vi "Do Main Action.vi"(8 "error in (no error)":errorcluster, 10 "AbstractData":refnum<class "AbstractData.lvclass">, 11 "Pipelined Actor in":refnum<class "Pipelined Actor.lvclass">) -> (0 "error out":errorcluster, 3 "Pipelined Actor out":refnum<class "Pipelined Actor.lvclass">)   [LabVIEW 2014, in "Pipelined Actor.lvlib" / "Pipelined Actor.lvclass"]
uses:
  Pipelined Actor.lvclass
  Model/Data/AbstractData/AbstractData.lvclass
  Pipelined Actor.lvclass/Pipelined Actor.ctl
  <vilib>/ActorFramework/Message Enqueuer/Message Priority.ctl
  Pipelined Actor Messages/Do Main Action Msg/Do Main Action Msg.lvclass/Do Main Action Msg.ctl
  <vilib>/ActorFramework/Message Enqueuer/Message Enqueuer.lvclass/Message Enqueuer.ctl
  <vilib>/ActorFramework/Message Enqueuer/Enqueue.vi
  <vilib>/ActorFramework/Message Priority Queue/Priority Enqueue.vi
  <vilib>/ActorFramework/Message Enqueuer/Message Enqueuer.lvclass
  Pipelined Actor Messages/Do Main Action Msg/Do Main Action Msg.lvclass
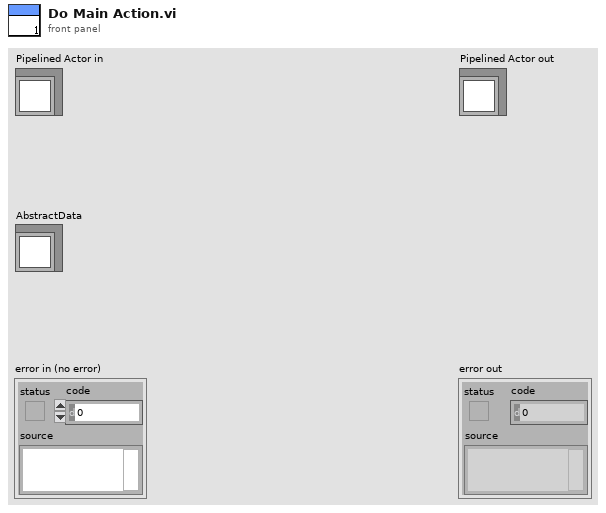
[diagram p1: front panel]
types:
  T1 = typedef "Actor Framework.lvlib/Message Enqueuer.lvclass/Message Priority.ctl" = enum16{"Low", "Normal", "High"}
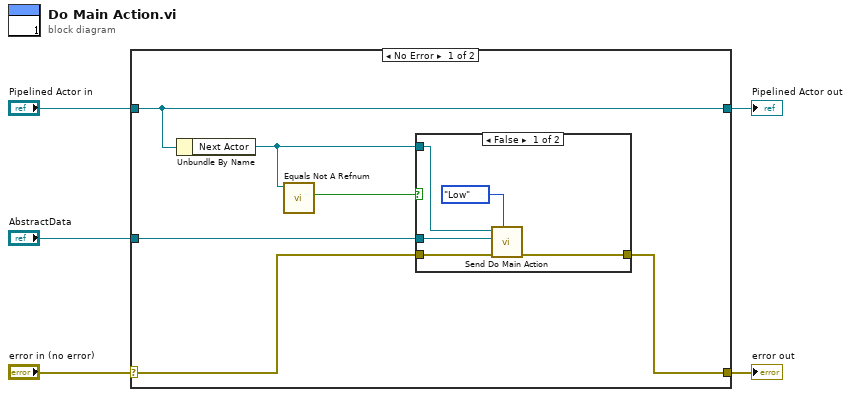
[diagram p0: block diagram]
diagram:
  n1 = case shown="No Error" "error in (no error)" {
    selector: "error in (no error)" -> [w7 w19]
    tunnel: [w6 w19] -> w4
    tunnel: [w11 w18] -> w2
    tunnel: "Pipelined Actor in" -> [w11 w18]
    tunnel: "AbstractData" -> [w8 _]
    frame No Error {
      n2 = Unbundle By Name(w11) -> ("Next Actor"=w9:refnum<class "Message Enqueuer.lvclass">)
      n3 = call <vilib>:"Equals Not A Refnum.vi"("Message Enqueuer"=w9) -> ("Not a refnum?"=w10:bool)  [unwired: 10 in]
      n4 = case shown="False" w10 {
        tunnel: w9 -> [w16 _]
        tunnel: w8 -> [w15 _]
        tunnel: w7 -> [w14 w17]
        tunnel: [w13 w17] -> w6
        frame False {
          n5 = call "Send Do Main Action.vi"("Message Priority (Normal)"=Message_Priority."Low", "error in (no error)"=w14, "AbstractData"=w15, "Message Enqueuer"=w16) -> ("error out"=w13:errorcluster)  [unwired: 6 in, 1 out]
        }
        frame True {
        }
      }
    }
    frame Error {
    }
  }
  "error out" <- w4
  "Pipelined Actor out" <- w2
